vi "niFpgaButterflyTemp_1Pipe.vi"(0 "x_r":fxp<+/-,16,1>, 1 "mult output type":fxp<+/-,16,1> format="%.16g", 2 "bf bullet type":fxp<+/-,32,16> format="%.21g", 5 "x_i":fxp<+/-,16,1>, 7 "y_r":fxp<+/-,16,1>, 9 "y_i":fxp<+/-,16,1>, 12 "tf_r":fxp<+/-,16,1>, 13 "tf_i":fxp<+/-,16,1>, 14 "first stage":bool) -> (4 "x_out_r":fxp<+/-,16,1>, 6 "x_out_i":fxp<+/-,16,1>, 8 "y_out_r":fxp<+/-,16,1>, 10 "y_out_i":fxp<+/-,16,1>)   [LabVIEW 2017]
uses:
  <vilib>/rvi/FXPMathLib/FxpMul/XNode/nifxpmath_Multiplier.xnode
  <vilib>/rvi/FXPMathLib/sim/FxpSim.dll
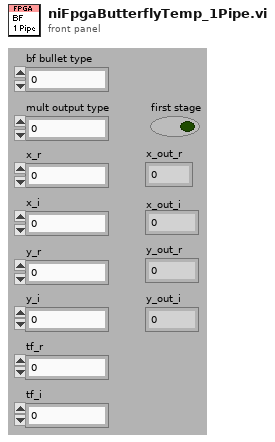
[diagram p1: front panel]
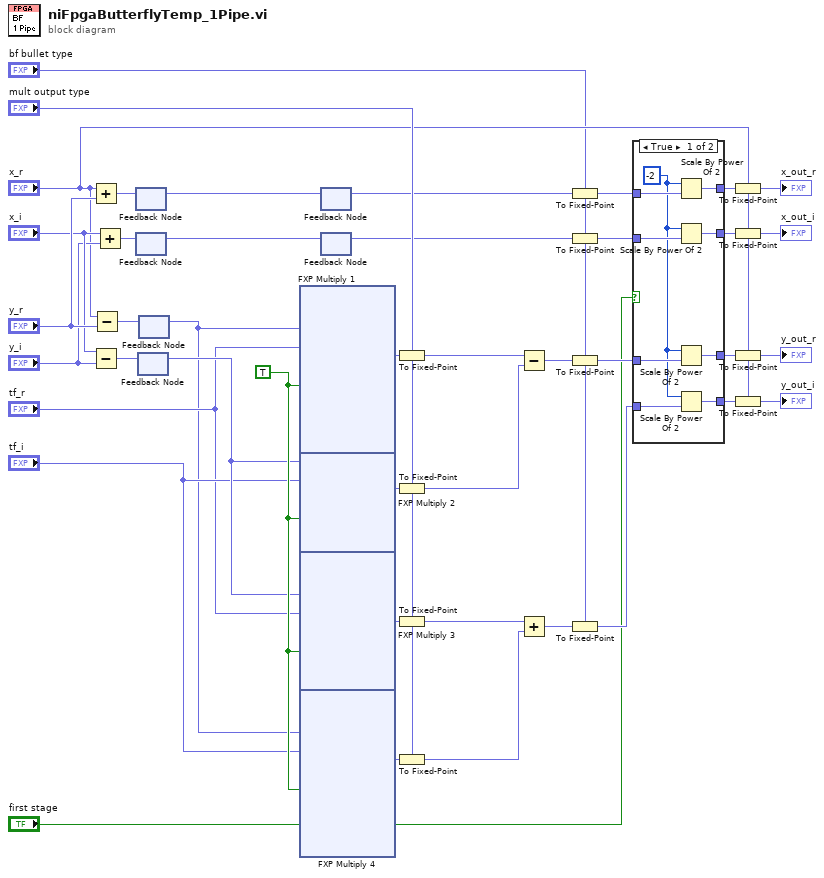
[diagram p0: block diagram]
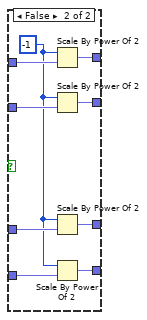
[diagram p2: hidden frame]
diagram:
  w32 = TRUE ("input valid")
  n1 = Add(x="x_r", y="y_r") -> (x+y=w27:fxp<+/-,17,2>)
  n2 = Subtract(x="x_i", y="y_i") -> (x-y=w41:fxp<+/-,17,2>)
  n3 = Subtract(x="x_r", y="y_r") -> (x-y=w42:fxp<+/-,17,2>)
  n4 = Add(x="x_i", y="y_i") -> (x+y=w26:fxp<+/-,17,2>)
  n5 = feedback-in #1(w27) -> ()
  n6 = feedback #1() -> (w33:fxp<+/-,17,2>)  [unwired: 1 out]
  n7 = feedback-in #2(w26) -> ()
  n8 = feedback #2() -> (w25:fxp<+/-,17,2>)  [unwired: 1 out]
  n9 = feedback-in #3(w41) -> ()
  n10 = feedback #3() -> (w31:fxp<+/-,17,2>)  [unwired: 1 out]
  n11 = feedback-in #4(w42) -> ()
  n12 = feedback #4() -> (w28:fxp<+/-,17,2>)  [unwired: 1 out]
  n13 = xnode "FXP Multiply 1"("x"=w28, "y"="tf_r", "input valid"=w32) -> ("x*y"=w17:fxp<+/-,33,3>)  [unwired: 1 in, 2 out]
  n14 = xnode "FXP Multiply 2"("x"=w31, "y"="tf_i", "input valid"=w32) -> ("x*y"=w20:fxp<+/-,33,3>)  [unwired: 1 in, 2 out]
  n15 = xnode "FXP Multiply 3"("x"=w31, "y"="tf_r", "input valid"=w32) -> ("x*y"=w22:fxp<+/-,33,3>)  [unwired: 1 in, 2 out]
  n16 = xnode "FXP Multiply 4"("x"=w28, "y"="tf_i", "input valid"=w32) -> ("x*y"=w24:fxp<+/-,33,3>)  [unwired: 1 in, 2 out]
  n17 = feedback-in #5(w33) -> ()
  n18 = feedback #5() -> (w12:fxp<+/-,17,2>)  [unwired: 1 out]
  n19 = feedback-in #6(w25) -> ()
  n20 = feedback #6() -> (w11:fxp<+/-,17,2>)  [unwired: 1 out]
  n21 = To Fixed-Point(fixed-point type="mult output type", number=w17) -> (fixed-point=w18:fxp<+/-,16,1>)
  n22 = To Fixed-Point(fixed-point type="mult output type", number=w20) -> (fixed-point=w19:fxp<+/-,16,1>)
  n23 = To Fixed-Point(fixed-point type="mult output type", number=w22) -> (fixed-point=w21:fxp<+/-,16,1>)
  n24 = To Fixed-Point(fixed-point type="mult output type", number=w24) -> (fixed-point=w23:fxp<+/-,16,1>)
  n25 = Subtract(x=w18, y=w19) -> (x-y=w13:fxp<+/-,17,2>)
  n26 = Add(x=w21, y=w23) -> (x+y=w14:fxp<+/-,17,2>)
  n27 = To Fixed-Point(fixed-point type="bf bullet type", number=w12) -> (fixed-point=w9:fxp<+/-,32,16>)
  n28 = To Fixed-Point(fixed-point type="bf bullet type", number=w11) -> (fixed-point=w8:fxp<+/-,32,16>)
  n29 = To Fixed-Point(fixed-point type="bf bullet type", number=w13) -> (fixed-point=w7:fxp<+/-,32,16>)
  n30 = To Fixed-Point(fixed-point type="bf bullet type", number=w14) -> (fixed-point=w6:fxp<+/-,32,16>)
  n31 = case shown="True" "first stage" {
    tunnel: [w51 w60] -> w5
    tunnel: [w50 w59] -> w4
    tunnel: [w49 w58] -> w3
    tunnel: [w48 w57] -> w2
    tunnel: w6 -> [w47 w56]
    tunnel: w7 -> [w46 w55]
    tunnel: w9 -> [w45 w54]
    tunnel: w8 -> [w44 w53]
    frame True {
      w43 = -2 ("n")
      n32 = Scale By Power Of 2(n=w43, x=w45) -> (x*2^n=w51:fxp<+/-,32,16>)
      n33 = Scale By Power Of 2(n=w43, x=w44) -> (x*2^n=w50:fxp<+/-,32,16>)
      n34 = Scale By Power Of 2(n=w43, x=w46) -> (x*2^n=w49:fxp<+/-,32,16>)
      n35 = Scale By Power Of 2(n=w43, x=w47) -> (x*2^n=w48:fxp<+/-,32,16>)
    }
    frame False {
      w52 = -1 ("n")
      n36 = Scale By Power Of 2(n=w52, x=w54) -> (x*2^n=w60:fxp<+/-,32,16>)
      n37 = Scale By Power Of 2(n=w52, x=w53) -> (x*2^n=w59:fxp<+/-,32,16>)
      n38 = Scale By Power Of 2(n=w52, x=w55) -> (x*2^n=w58:fxp<+/-,32,16>)
      n39 = Scale By Power Of 2(n=w52, x=w56) -> (x*2^n=w57:fxp<+/-,32,16>)
    }
  }
  n40 = To Fixed-Point(fixed-point type="x_r", number=w5) -> (fixed-point=→"x_out_r":fxp<+/-,16,1>)
  n41 = To Fixed-Point(fixed-point type="x_r", number=w4) -> (fixed-point=→"x_out_i":fxp<+/-,16,1>)
  n42 = To Fixed-Point(fixed-point type="x_r", number=w3) -> (fixed-point=→"y_out_r":fxp<+/-,16,1>)
  n43 = To Fixed-Point(fixed-point type="x_r", number=w2) -> (fixed-point=→"y_out_i":fxp<+/-,16,1>)
